vi "修改-探头报警值-30.vi"(6 "VI引用句柄":refnum<vi>, 7 "修改模式":enum16{"全部限值", "一级限值", "二级限值"}(ring), 8 "VISA资源名称":refnum<visa-resource-name>, 9 "限值 i":T1(array[cluster]), 10 "探头地址":i32[](array[numeric]), 11 "实时数据列表":refnum<vi>) -> (3 "限值 o":T1(array[cluster]))   [LabVIEW 2017]
panel:
  in  "探头限值":enum16{"一级限值", "二级限值"}(ring)
  in  "限值2":sgl=0.5 min=0 max=6553.6 format="%#.1f"
  in  "单位2":enum8{"uSv/h", "mSv/h"}(ring)
  in  "取消按钮":bool
  in  "确定按钮":bool
  in  "限值1":sgl=0.5 min=0 max=6553.6 format="%#.1f"
  in  "单位1":enum8{"uSv/h", "mSv/h"}(ring)
  out "提示语":string
  out "引用-暂停发送":refnum<vi>
  # "剂量率限值"
  # "一级报警限值"
  # "二级报警限值"
  # "限值分配"
  # "设为探头报警值"
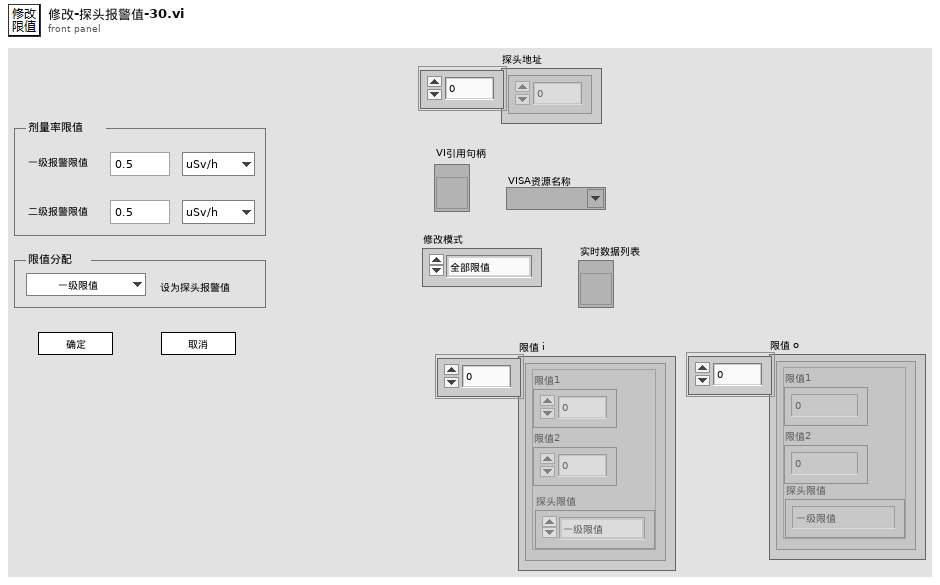
[diagram p1: front panel]
types:
  T1 = cluster{"限值1":dbl, "限值2":dbl, "探头限值":enum16{"一级限值", "二级限值"}}[]
  T2 = cluster{"限值1":dbl, "限值2":dbl, "探头限值":enum16{"一级限值", "二级限值"}}
  T3 = enum32{"Invalid", "Standard", "Closed", "Hidden", "Minimized", "Maximized"}
  T4 = enum8{"Enabled", "Disabled", "Disabled and Grayed Out"}
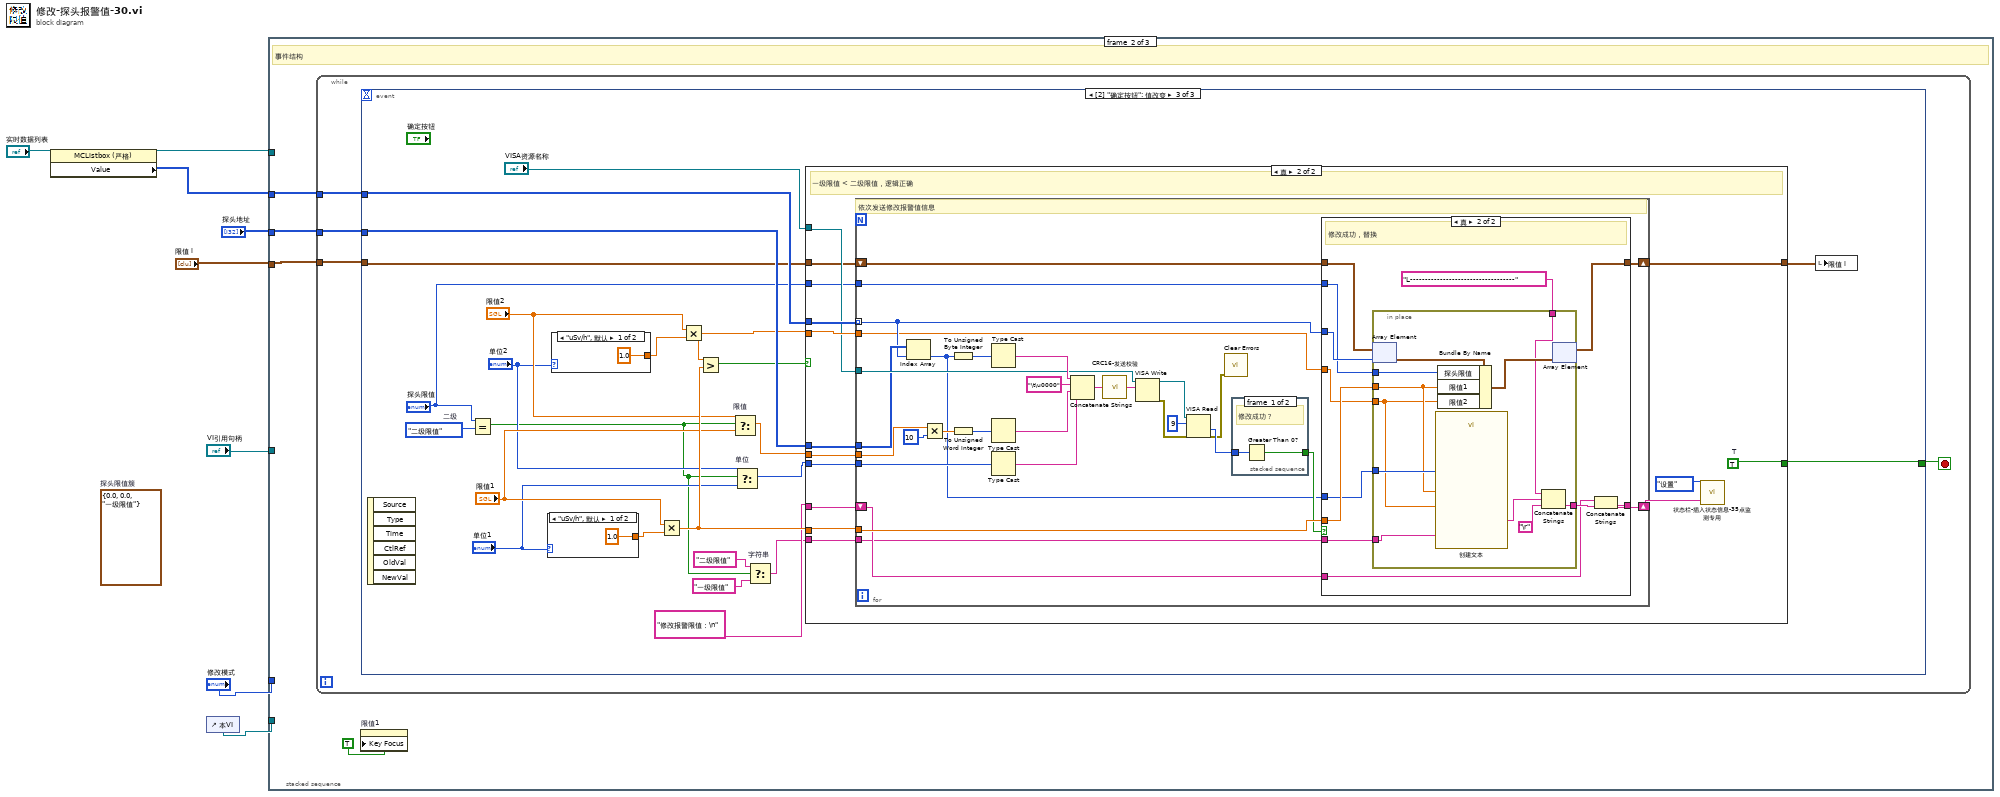
[diagram p0: block diagram]
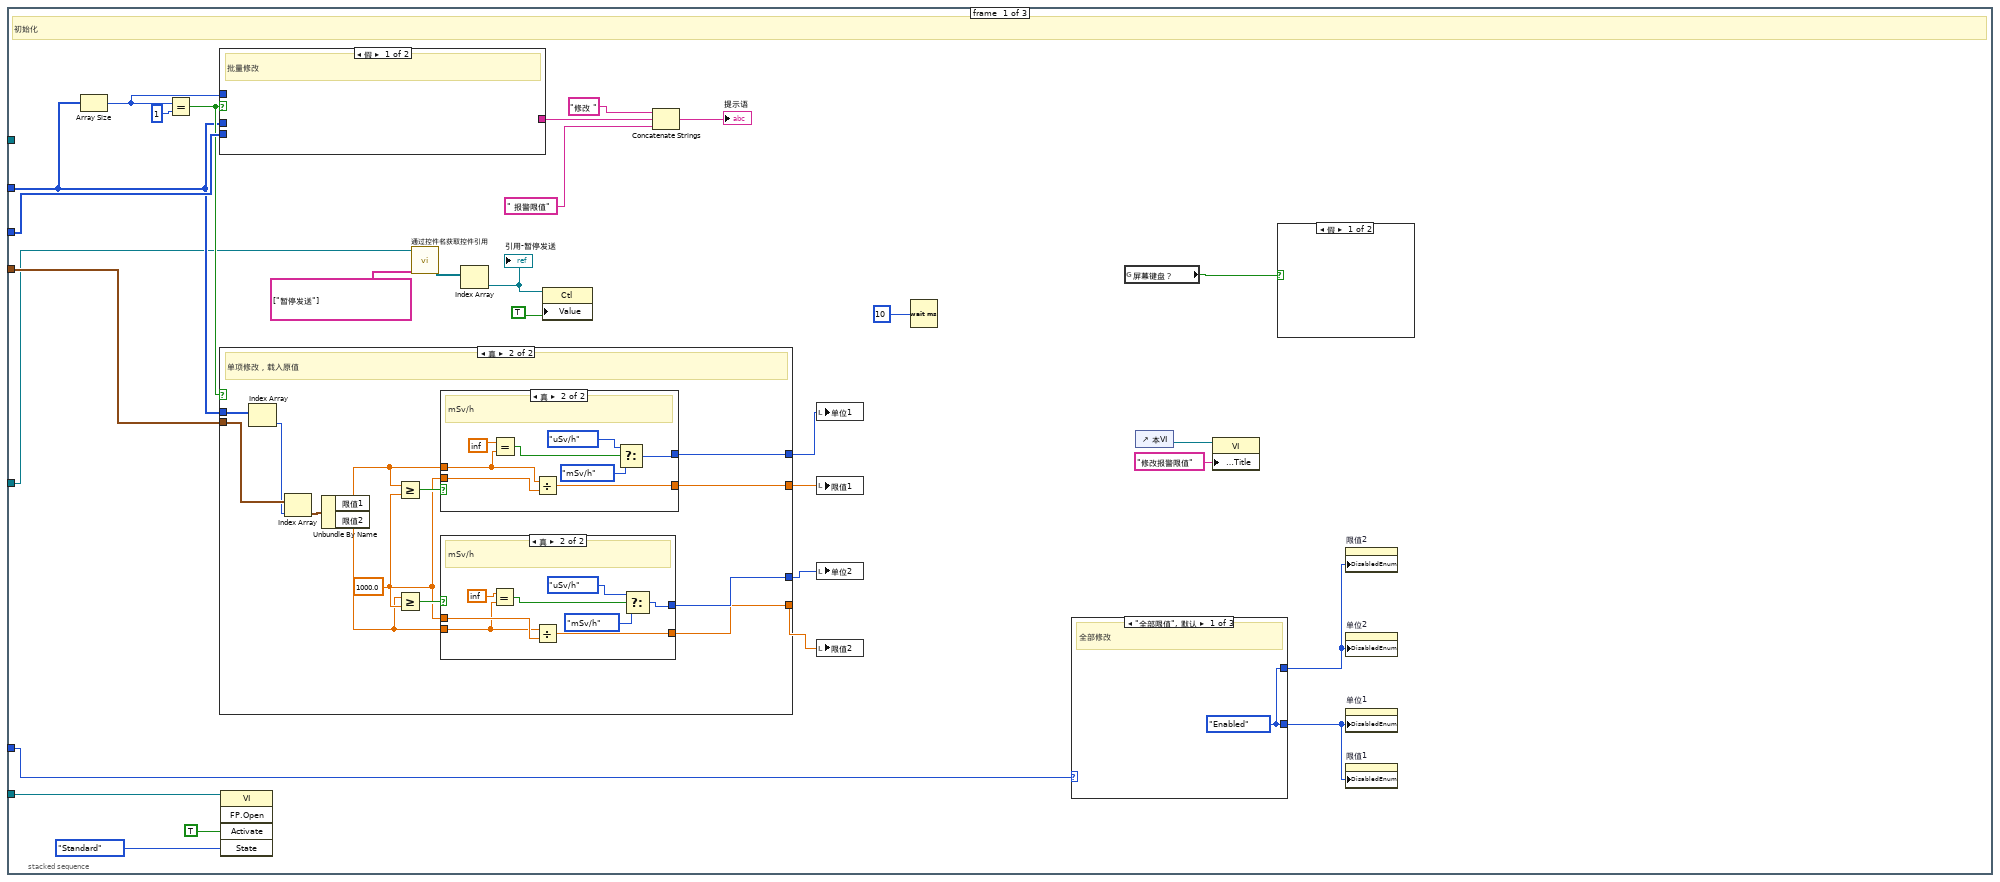
[diagram p2: hidden frame]
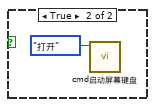
[diagram p3: hidden frame]
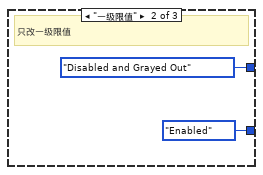
[diagram p4: hidden frame]
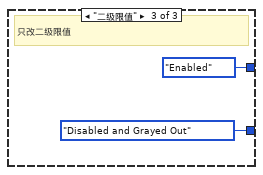
[diagram p5: hidden frame]
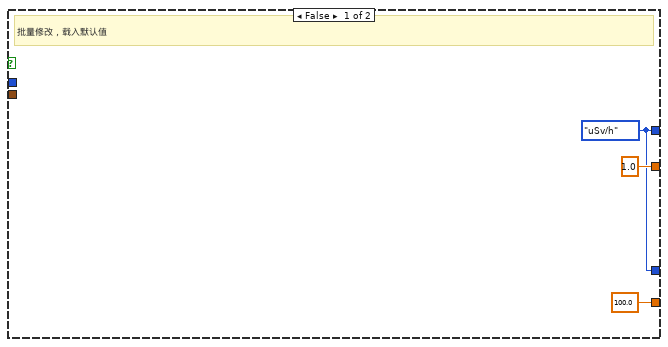
[diagram p6: hidden frame]
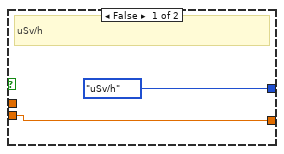
[diagram p7: hidden frame]
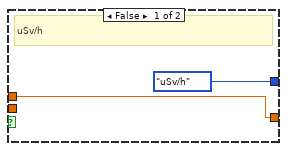
[diagram p8: hidden frame]
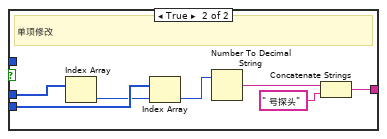
[diagram p9: hidden frame]
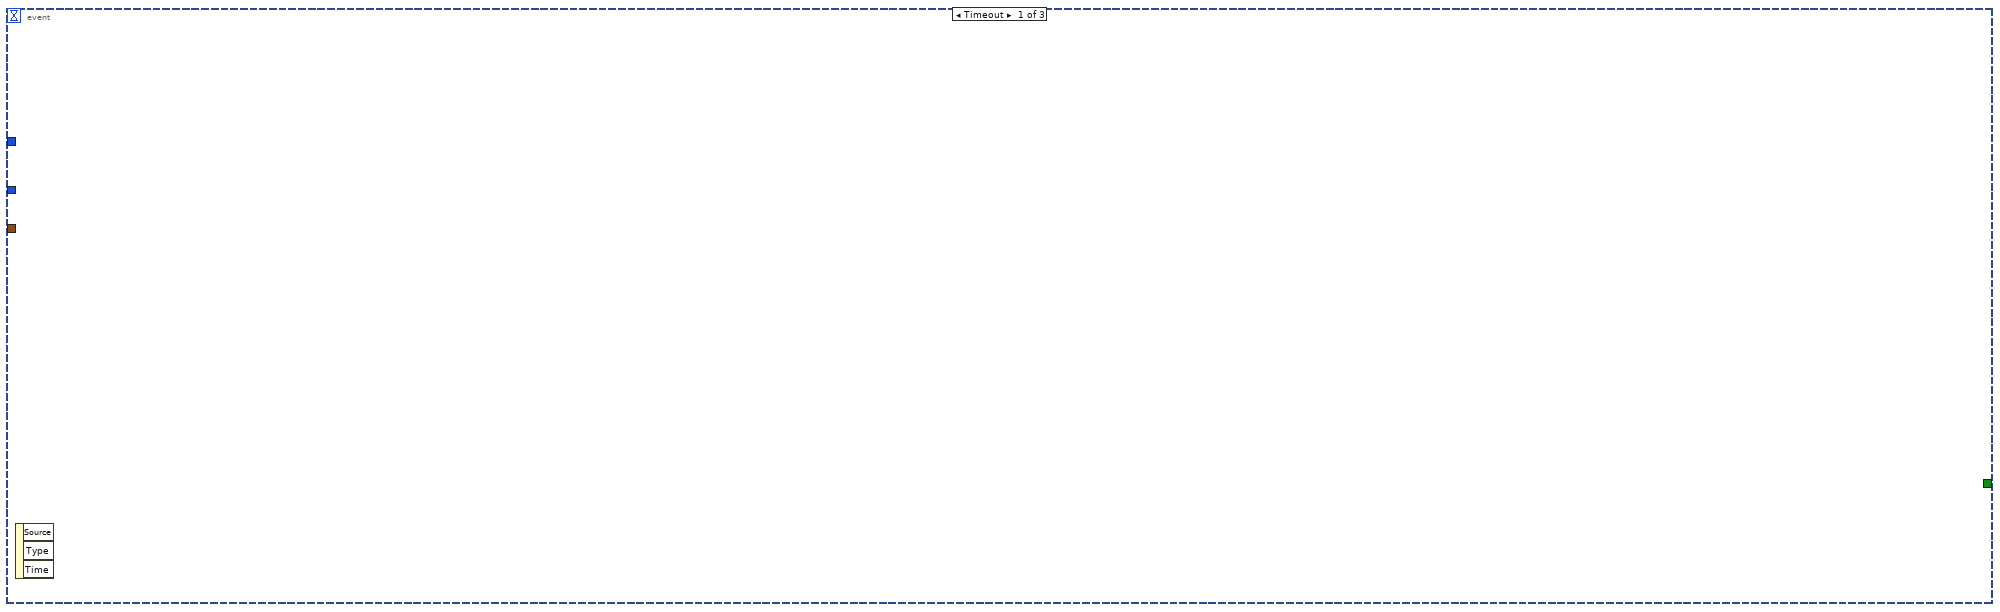
[diagram p10: hidden frame]
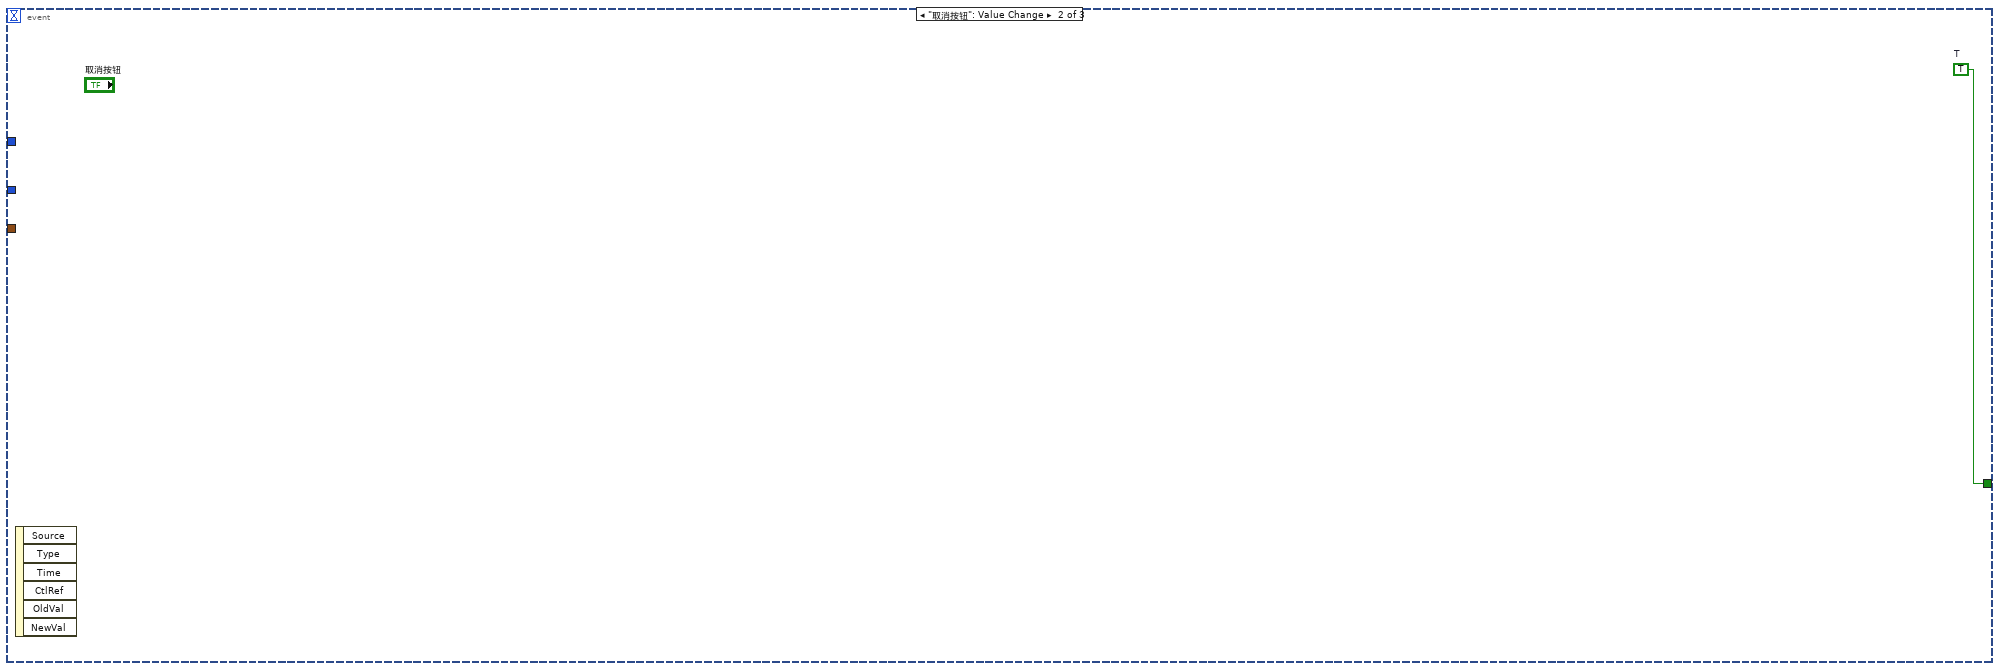
[diagram p11: hidden frame]
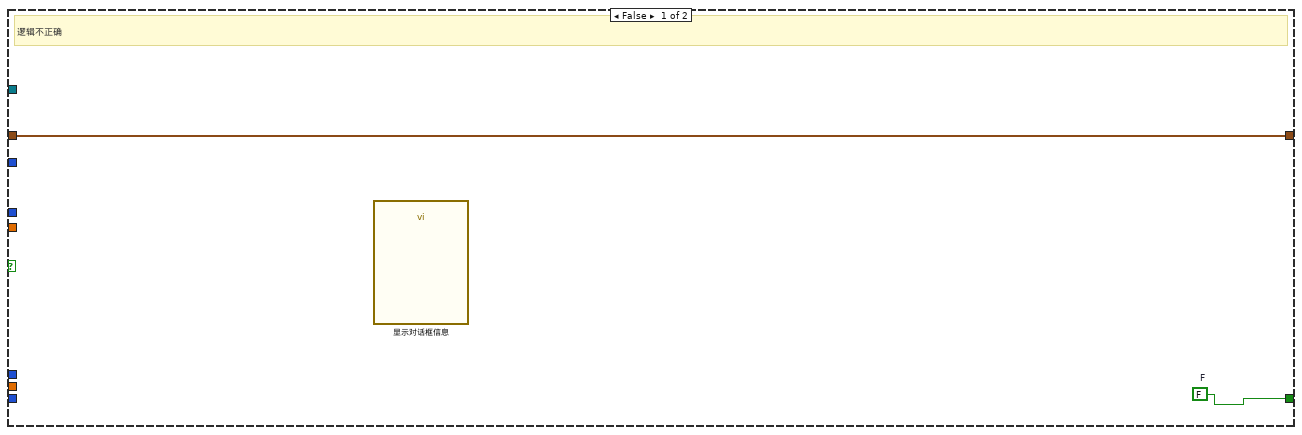
[diagram p12: hidden frame]
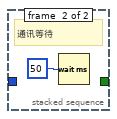
[diagram p14: hidden frame]
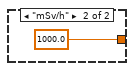
[diagram p15: hidden frame]
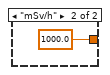
[diagram p16: hidden frame]
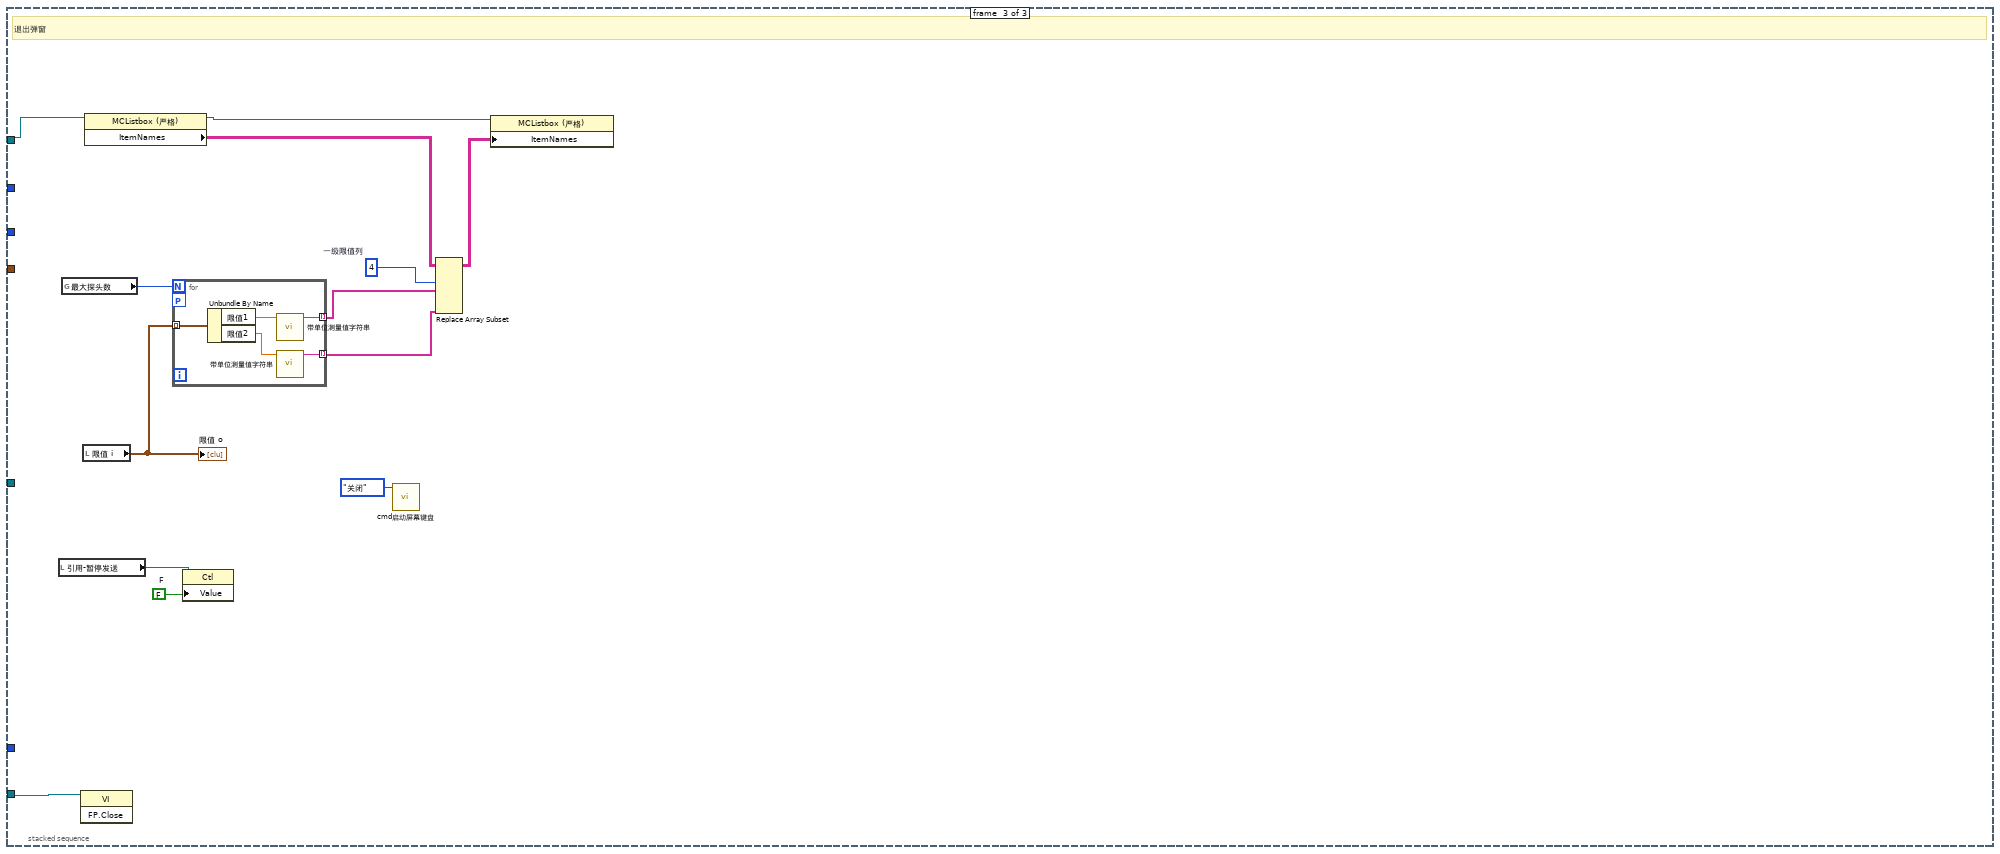
[diagram p17: hidden frame]
diagram:
  (unwired) T2 {"限值1"=0.0, "限值2"=0.0, "探头限值"=enum."一级限值"}  # 探头限值簇
  n1 = property class="MCListbox (严格)"(reference="实时数据列表") -> (reference out=w1:refnum<vi>, "Value"=w2:i32[])  [unwired: 1 in, 1 out]
  n2 = control-ref of="本VI"() -> (w7:refnum<vi>)
  n3 = stacked-sequence {
    tunnel: w2 -> [w26 w90 _]
    tunnel: "VI引用句柄" -> [w15 _ _]
    tunnel: w7 -> [w32 _ w210]
    tunnel: "探头地址" -> [w30 w89 _]
    tunnel: "限值 i" -> [w21 w88 _]
    tunnel: "修改模式" -> [w20 _ _]
    tunnel: w1 -> [_ _ w206]
    frame #0 {
      # "初始化"
      n4 = Array Size(array=w26) -> (size(s)=w29:i32)
      n5 = Equal?(x=w29, y=1) -> (x = y?=w27:bool)
      n6 = case shown="假" w27 {
        tunnel: w30 -> [_ w86]
        tunnel: w26 -> [_ w85]
        tunnel: w29 -> [_ _]
        tunnel: [_ w80] -> w28
        frame False {
          # "批量修改"
        }
        frame True {
          # "单项修改"
          n7 = Index Array(array=w85) -> (element=w84:i32)  [unwired: 1 in]
          n8 = Index Array(array=w86, index=w84) -> (element=w83:i32)
          n9 = Number To Decimal String(number=w83) -> (decimal integer string=w82:string)  [unwired: 1 in]
          n10 = Concatenate Strings(w82, " 号探头" ("字符串")) -> (w80:string)
        }
      }
      n11 = case shown="真" w27 {
        tunnel: w21 -> [_ w51]
        tunnel: w26 -> [_ w59]
        tunnel: [1.0 ("数值输入控件") w55] -> w25
        tunnel: [w45 w54] -> w24
        tunnel: [w45 w53] -> w23
        tunnel: [100.0 ("数值输入控件") w52] -> w22
        frame False {
          w45 = enum8{"uSv/h", "mSv/h"}."uSv/h" ("单位1")
          # "批量修改，载入默认值"
        }
        frame True {
          w56 = 1000.0 ("y")
          # "单项修改，载入原值"
          n12 = Index Array(array=w59) -> (element=w50:i32)  [unwired: 1 in]
          n13 = Index Array(array=w51, index=w50) -> (element=w49:T2)
          n14 = Unbundle By Name(w49) -> ("限值1"=w48:dbl, "限值2"=w47:dbl)
          n15 = Greater Or Equal?(x=w48, y=w56) -> (x >= y?=w57:bool)
          n16 = Greater Or Equal?(x=w47, y=w56) -> (x >= y?=w58:bool)
          n17 = case shown="真" w57 {
            tunnel: w48 -> [w70 w77]
            tunnel: w56 -> [_ w79]
            tunnel: [w70 w78] -> w55
            tunnel: [enum8{"uSv/h", "mSv/h"}."uSv/h" ("单位1") w72] -> w54
            frame False {
              # "uSv/h"
            }
            frame True {
              # "mSv/h"
              n18 = Equal?(x=inf, y=w77) -> (x = y?=w75:bool)
              n19 = Divide(x=w77, y=w79) -> (x/y=w78:dbl)
              n20 = Select(t=enum8{"uSv/h", "mSv/h"}."uSv/h" ("单位1"), s=w75, f=enum8{"uSv/h", "mSv/h"}."mSv/h" ("单位1")) -> (s? t:f=w72:enum8{"uSv/h", "mSv/h"})
            }
          }
          n21 = case shown="真" w58 {
            tunnel: w47 -> [w60 w66]
            tunnel: w56 -> [_ w69]
            tunnel: [enum8{"uSv/h", "mSv/h"}."uSv/h" ("单位1") w62] -> w53
            tunnel: [w60 w68] -> w52
            frame False {
              # "uSv/h"
            }
            frame True {
              # "mSv/h"
              n22 = Equal?(x=inf, y=w66) -> (x = y?=w65:bool)
              n23 = Divide(x=w66, y=w69) -> (x/y=w68:dbl)
              n24 = Select(t=enum8{"uSv/h", "mSv/h"}."uSv/h" ("单位1"), s=w65, f=enum8{"uSv/h", "mSv/h"}."mSv/h" ("单位1")) -> (s? t:f=w62:enum8{"uSv/h", "mSv/h"})
            }
          }
        }
      }
      n25 = invoke class="VI" method="FP.Open"(reference=w32, "Activate"=TRUE ("激活？"), "State"=T3."Standard" ("状态")) -> ()  [unwired: 2 in, 5 out]
      n26 = call "通过控件名获取控件引用.vi"("控件名数组"=string[] ["暂停发送"], "VI引用"=w15) -> ("控件引用输出"=w16:refnum<vi>[])  [unwired: 7 in, 2 out]
      n27 = Index Array(array=w16) -> (element=w13:refnum<vi>)  [unwired: 1 in]
      "引用-暂停发送" <- w13
      n28 = property class="Ctl"(reference=w13, "Value"=TRUE ("T")) -> ()  [unwired: 1 in, 2 out]
      n29 = Concatenate Strings("修改 " ("字符串"), w28, " 报警限值" ("字符串")) -> (→"提示语":string)
      n30 = local write "单位1"(w24) -> ()
      n31 = local write "限值1"(w25) -> ()
      n32 = local write "单位2"(w23) -> ()
      n33 = local write "限值2"(w22) -> ()
      n34 = Wait (ms)(milliseconds to wait=u32 10 ("等待时间（毫秒）")) -> ()  [unwired: 1 out]
      n35 = case shown="\"全部限值\", 默认" w20 {
        tunnel: [w39 T4."Enabled" ("禁用") T4."Disabled and Grayed Out" ("禁用")] -> w19
        tunnel: [w39 T4."Disabled and Grayed Out" ("禁用") T4."Enabled" ("禁用")] -> w18
        frame "全部限值", Default {
          w39 = T4."Enabled" ("禁用")
          # "全部修改"
        }
        frame "一级限值" {
          # "只改一级限值"
        }
        frame "二级限值" {
          # "只改二级限值"
        }
      }
      n36 = global read "全局变量-35点监测.vi" "屏幕键盘？"() -> (w11:bool)
      n37 = control-ref of="本VI"() -> (w10:refnum<vi>)
      n38 = property class="VI"(reference=w10, "Front Panel.Title"="修改报警限值" ("前面板窗口:标题")) -> ()  [unwired: 1 in, 2 out]
      n39 = case shown="假" w11 {
        frame False {
        }
        frame True {
          n40 = call "cmd启动屏幕键盘.vi"("软键盘开关"=enum16{"关闭", "打开"}."打开") -> ()  [unwired: 9 in, 2 out]
        }
      }
      n41 = property on="限值2" class="DigNum (严格)"("DisabledEnum"=w18) -> ()  [unwired: 2 in, 2 out]
      n42 = property on="单位2" class="Enum (严格)"("DisabledEnum"=w18) -> ()  [unwired: 2 in, 2 out]
      n43 = property on="单位1" class="Enum (严格)"("DisabledEnum"=w19) -> ()  [unwired: 2 in, 2 out]
      n44 = property on="限值1" class="DigNum (严格)"("DisabledEnum"=w19) -> ()  [unwired: 2 in, 2 out]
    }
    frame #1 {
      # "事件结构"
      n45 = while {
        tunnel: w90 -> [w93]
        tunnel: w89 -> [w92]
        tunnel: w88 -> [w91]
        stop <- w94 stop-if-true
        n46 = event shown="[2] \"确定按钮\": 值改变" {
          selector: _ -> [_ _ _]
          dyn-events: _ -> [_ _ _]
          timeout: _ -> [_ _ _]
          tunnel: [_ w95 w114] -> w94
          tunnel: w93 -> [_ _ w119]
          tunnel: w92 -> [_ _ w118]
          tunnel: w91 -> [_ _ w116]
          event Timeout {
            n47 = event-data() -> ()  [unwired: 1 in, 3 out]
          }
          event "取消按钮": Value Change {
            w95 = TRUE  # T
            n48 = event-data() -> ()  [unwired: 1 in, 6 out]
          }
          event "确定按钮": Value Change {
            w107 = enum16{"一级限值", "二级限值"}."二级限值"  # 二级
            n49 = event-data() -> ()  [unwired: 1 in, 6 out]
            n50 = Equal?(x="探头限值", y=w107) -> (x = y?=w99:bool)
            n51 = case shown="\"uSv/h\", 默认" "单位1" {
              tunnel: [sgl 1.0 ("探头报警值") sgl 1000.0 ("探头报警值")] -> w113
              frame "uSv/h", Default {
              }
              frame "mSv/h" {
              }
            }
            n52 = case shown="\"uSv/h\", 默认" "单位2" {
              tunnel: [sgl 1.0 ("探头报警值") sgl 1000.0 ("探头报警值")] -> w112
              frame "uSv/h", Default {
              }
              frame "mSv/h" {
              }
            }
            n53 = Multiply(x="限值1", y=w113) -> (x*y=w109:sgl)
            n54 = Multiply(x="限值2", y=w112) -> (x*y=w110:sgl)
            n55 = Greater?(x=w110, y=w109) -> (0:w111:bool)
            n56 = Select "限值"(t="限值2", s=w99, f="限值1") -> (s? t:f=w101:sgl)
            n57 = Select "单位"(t="单位2", s=w99, f="单位1") -> (s? t:f=w102:enum8{"uSv/h", "mSv/h"})
            n58 = Select "字符串"(t="二级限值", s=w99, f="一级限值") -> (s? t:f=w96:string)
            n59 = case shown="真" w111 {
              tunnel: w119 -> [_ w136]
              tunnel: w109 -> [_ w135]
              tunnel: w101 -> [_ w134]
              tunnel: w102 -> [_ w133]
              tunnel: w118 -> [_ w132]
              tunnel: w110 -> [_ w131]
              tunnel: "VISA资源名称" -> [_ w130]
              tunnel: w116 -> [w120 w129]
              tunnel: [w120 w128] -> w115
              tunnel: [w121 w127] -> w114
              tunnel: "修改报警限值：\n" -> [_ w124]
              tunnel: "探头限值" -> [_ w123]
              tunnel: w96 -> [_ w122]
              frame False {
                w121 = FALSE  # F
                # "逻辑不正确"
                n60 = call "显示对话框信息"() -> ()  [unwired: 10 in, 2 out]
              }
              frame True {
                w127 = TRUE  # T
                # "一级限值 < 二级限值，逻辑正确"
                n61 = for {
                  tunnel: w130 -> [w157]
                  tunnel: w136 -> [w147] mode=indexing
                  tunnel: w132 -> [w155]
                  tunnel: w134 -> [w154]
                  tunnel: w133 -> [w153]
                  tunnel: w135 -> [w152]
                  tunnel: w131 -> [w145]
                  shift-right: [w143] -> w128
                  shift-left: w129 -> [w144]
                  shift-right: [w140] -> w125
                  shift-left: w124 -> [w139]
                  tunnel: w123 -> [w138]
                  tunnel: w122 -> [w137]
                  # "依次发送修改报警值信息"
                  n62 = Index Array(array=w155, index=w147) -> (element=w141:i32)
                  n63 = Multiply(x=w154, y=10) -> (x*y=w163:sgl)
                  n64 = To Unsigned Byte Integer(number=w141) -> (unsigned 8bit integer=w156:u8)
                  n65 = To Unsigned Word Integer(number=w163) -> (unsigned 16bit integer=w162:u16)
                  n66 = Type Cast(x=w156) -> (*(type *) &x=w158:string)  [unwired: 1 in]
                  n67 = Type Cast(x=w162) -> (*(type *) &x=w161:string)  [unwired: 1 in]
                  n68 = Type Cast(x=w153) -> (*(type *) &x=w159:string)  [unwired: 1 in]
                  n69 = Concatenate Strings(w158, "\t\u0000", w161, w159) -> (w166:string)
                  n70 = call "CRC16-发送校验.vi"("净数据"=w166) -> ("完整输出"=w160:string)
                  n71 = VISA Write(VISA resource name=w157, write buffer=w160) -> (VISA resource name out=w150:refnum<visa-resource-name>, error out=w151:errorcluster)  [unwired: 1 in, 1 out]
                  n72 = VISA Read(VISA resource name=w150, byte count=u32 9 ("字节总数"), error in (no error)=w151) -> (return count=w148:u32, error out=w142:errorcluster)  [unwired: 2 out]
                  n73 = call <vilib>:"Clear Errors.vi"("error in (no error)"=w142) -> ()  [unwired: 5 in, 2 out]
                  n74 = stacked-sequence {
                    tunnel: w148 -> [w192 _]
                    tunnel: [w191 _] -> w146
                    frame #0 {
                      # "修改成功？"
                      n75 = Greater Than 0?(x=w192) -> (x > 0?=w191:bool)
                    }
                    frame #1 {
                      # "通讯等待"
                      n76 = Wait (ms)(milliseconds to wait=u32 50 ("等待时间（毫秒）")) -> ()  [unwired: 1 out]
                    }
                  }
                  n77 = case shown="真" w146 {
                    tunnel: w152 -> [_ w178]
                    tunnel: w147 -> [_ w175]
                    tunnel: w145 -> [_ w177]
                    tunnel: w144 -> [w167 w179]
                    tunnel: [w167 w176] -> w143
                    tunnel: w141 -> [_ w174]
                    tunnel: [_ w172] -> w140
                    tunnel: w139 -> [_ w171]
                    tunnel: w138 -> [_ w169]
                    tunnel: w137 -> [_ w168]
                    frame False {
                      # "未成功，不替换"
                    }
                    frame True {
                      # "修改成功，替换"
                      n78 = in-place {
                        in-place-border: w178 -> [w187]
                        in-place-border: w177 -> [w186]
                        in-place-border: w174 -> [w188]
                        in-place-border: [w184] -> w173
                        in-place-border: "L-----------------------------------" ("字符串") -> [w182]
                        in-place-border: w169 -> [w181]
                        in-place-border: w168 -> [w180]
                        n79 = in-place-array #1(w179, w175) -> (w189:T2)
                        n80 = call "创建文本"("探头限值分配"=w180, "编号"=w188, "一级"=w187, "二级"=w186) -> ("Result"=w185:string)  [unwired: 10 in, 1 out]
                        n81 = Bundle By Name(cluster=w189, "探头限值"=w181, "限值1"=w187, "限值2"=w186) -> (w190:T2)
                        n82 = Concatenate Strings(w182, w185, "\r") -> (w184:string)
                        n83 = in-place-array #1(w190) -> (w176:T1)  [unwired: 1 out]
                      }
                      n84 = Concatenate Strings(w171, w173) -> (w172:string)
                    }
                  }
                }
                n85 = call "状态栏-插入状态信息-35点监测专用.vi"("消息内容"=w125, "状态类型"=enum16{"全部", "报警", "通信", "设置"}."设置") -> ()  [unwired: 10 in]
              }
            }
            n86 = local write "限值 i"(w115) -> ()
          }
        }
      }
      n87 = property on="限值1" class="DigNum (严格)"("Key Focus"=TRUE ("键选中")) -> ()  [unwired: 2 in, 2 out]
    }
    frame #2 {
      w202 = 4  # 一级限值列
      w209 = FALSE  # F
      # "退出弹窗"
      n88 = local read "引用-暂停发送"() -> (w208:refnum<vi>)
      n89 = global read "全局变量-35点监测.vi" "最大探头数"() -> (w199:i32)
      n90 = invoke class="VI" method="FP.Close"(reference=w210) -> ()  [unwired: 2 in, 3 out]
      n91 = local read "限值 i"() -> (w207:T1)
      "限值 o" <- w207
      n92 = property class="MCListbox (严格)"(reference=w206) -> (reference out=w205:refnum<vi>, "ItemNames"=w204:string[][])  [unwired: 1 in, 1 out]
      n93 = for {
        N: w199 -> [_]
        tunnel: w207 -> [w215] mode=indexing
        workers-P: _ -> [_]
        tunnel: [w212] -> w201 mode=indexing
        tunnel: [w211] -> w200 mode=indexing
        n94 = Unbundle By Name(w215) -> ("限值1"=w214:dbl, "限值2"=w213:dbl)
        n95 = call "带单位测量值字符串.vi"("测量值"=w214) -> ("结果"=w212:string)  [unwired: 10 in]
        n96 = call "带单位测量值字符串.vi"("测量值"=w213) -> ("结果"=w211:string)  [unwired: 10 in]
      }
      n97 = property class="Ctl"(reference=w208, "Value"=w209) -> ()  [unwired: 1 in, 2 out]
      n98 = call "cmd启动屏幕键盘.vi"("软键盘开关"=enum16{"关闭", "打开"}."关闭") -> ()  [unwired: 9 in, 2 out]
      n99 = Replace Array Subset(array=w204, new element #1=w201, index (col) #1=w202, new element #2=w200) -> (w203:string[][])  [unwired: 3 in]
      n100 = property class="MCListbox (严格)"(reference=w205, "ItemNames"=w203) -> ()  [unwired: 1 in, 2 out]
    }
  }
